vi "OAT Ideal Hilbert Transformer Response.vi"(9 "fc":dbl format="%.2f", 10 "fs":dbl=1.0 format="%.2f", 11 "N":i32=16) -> (3 "coef":dbl[](array[numeric]) format="%.2f")   [LabVIEW 2017, in "SoundVib_Resampling.lvlib"]
uses:
  <vilib>/addons/Sound and Vibration/Order Analysis/Resample Order Tracking/SoundVib_Resampling.lvlib
  <vilib>/Analysis/1siggen.llb/Ramp Pattern by Samples.vi
  <vilib>/Analysis/NI_AALBase.lvlib
panel:
  out "Waveform Graph":dbl[](graph)
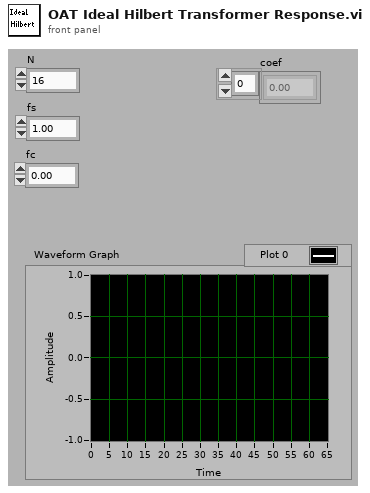
[diagram p1: front panel]
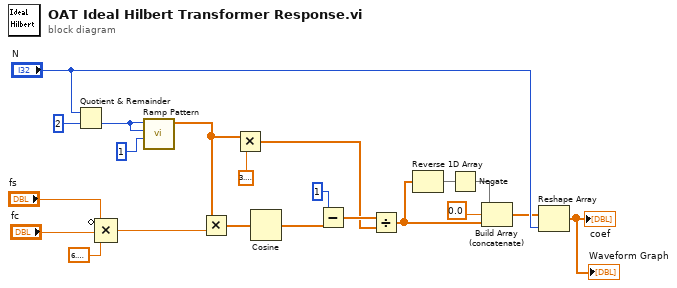
[diagram p0: block diagram]
diagram:
  n1 = Quotient & Remainder(x="N", y=2) -> (floor(x/y)=w4:i32)  [unwired: 1 out]
  n2 = Compound Arithmetic op=MULTIPLY(invert "fs", "fc", 6.283185307179586) -> (w17:dbl)
  n3 = call-poly <vilib>:"Ramp Pattern.vi"("start"=1, "end"=w4, "samples"=w4) -> ("Ramp Pattern"=w13:dbl[])  [unwired: 7 in, 1 out]
  n4 = Multiply(x=w13, y=w17) -> (x*y=w16:dbl[])
  n5 = Multiply(x=w13, y=3.141592653589793) -> (x*y=w10:dbl[])
  n6 = Cosine(x=w16) -> (cos(x)=w15:dbl[])
  n7 = Subtract(x=1, y=w15) -> (x-y=w11:dbl[])
  n8 = Divide(x=w11, y=w10) -> (x/y=w7:dbl[])
  n9 = Reverse 1D Array(array=w7) -> (reversed array=w9:dbl[])
  n10 = Negate(x=w9) -> (-x=w8:dbl[])
  n11 = Build Array (concatenate)(w8, 0.0, w7) -> (w2:dbl[])
  n12 = Reshape Array(w2, "N") -> (→"coef" →"Waveform Graph":dbl[])
